vi "example_00_architecture.vi"() -> ()   [LabVIEW 2015, in "lv-recipe-machine.lvlib"]
uses:
  lv-recipe-machine.lvlib
  public/_controls/mode.ctl
  public/_controls/manual_state.ctl
  public/_controls/automatic_state.ctl
panel:
  out "step_elapsed_time":dbl
  out "recipe_elapsed_time":dbl
  out "automatic_state":T1
  out "manual_state":T2
  out "mode 2":T3
  out "step":string
  out "data":variant
  in  "mode":T3
  in  "update_mode":bool
  out "error out":errorcluster
  in  "stop":bool
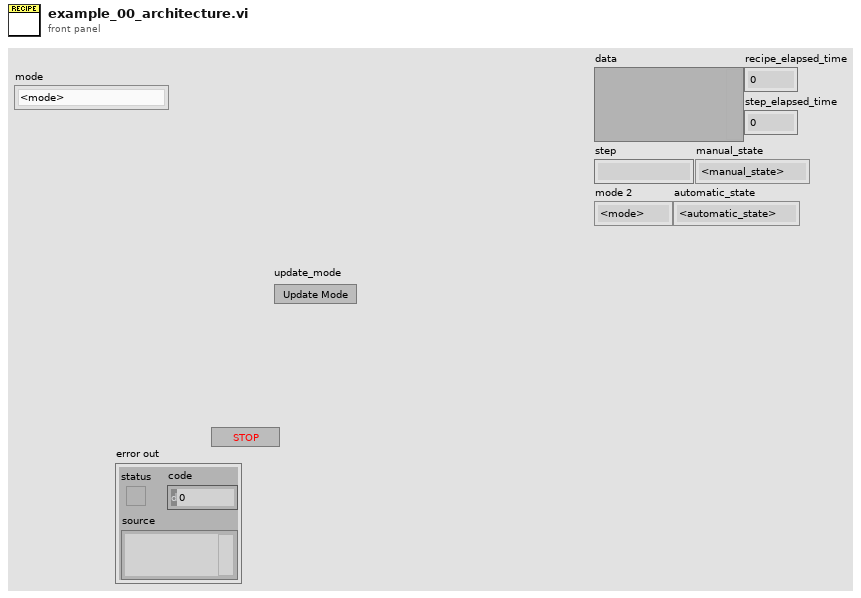
[diagram p1: front panel]
types:
  T1 = typedef "lv-recipe-machine.lvlib/automatic_state.ctl" = enum16{"<automatic_state>", "failed", "idle", "running", "paused", "stopped", "<null>"}
  T2 = typedef "lv-recipe-machine.lvlib/manual_state.ctl" = enum16{"<manual_state>", "failed", "action", "running", "idle", "<null>"}
  T3 = typedef "lv-recipe-machine.lvlib/mode.ctl" = enum16{"<mode>", "manual", "automatic", "<null>"}
  T4 = cluster{"change_out":refnum<event-registration>, "status_event_registration":refnum<event-registration>}
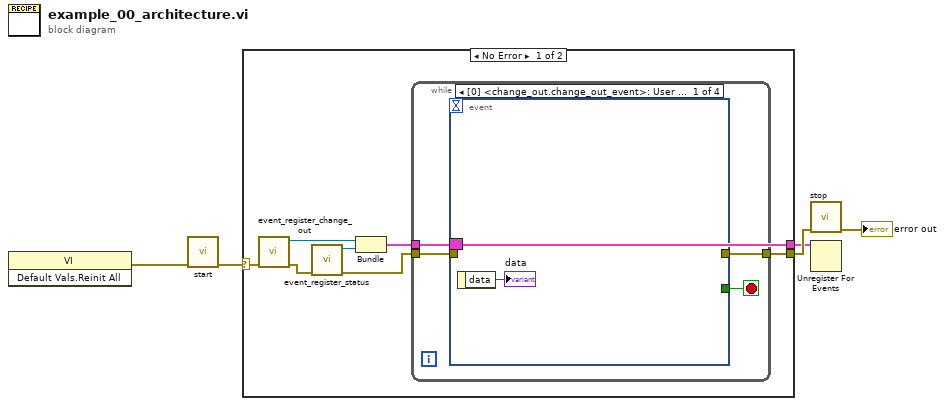
[diagram p0: block diagram]
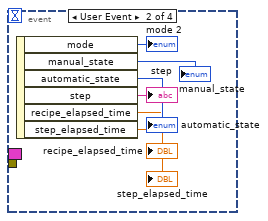
[diagram p2: hidden frame]
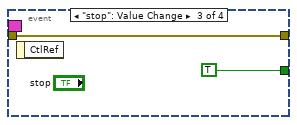
[diagram p3: hidden frame]
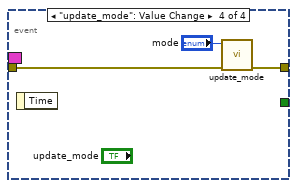
[diagram p4: hidden frame]
diagram:
  n1 = invoke class="VI" method="Default Vals.Reinit All"() -> (error out=w4:errorcluster)  [unwired: 3 in, 2 out]
  n2 = call "start.vi"("error in (no error)"=w4) -> ("error out"=w3:errorcluster)  [unwired: 10 in]
  n3 = case shown="No Error" w3 {
    selector: w3 -> [w8 w29]
    tunnel: [w12 w29] -> w5
    tunnel: [w9 _] -> w2
    frame No Error {
      n4 = call "event_register_change_out.vi"("error in (no error)"=w8) -> ("error out"=w7:errorcluster, "change_out"=w10:refnum<event-registration>)  [unwired: 9 in]
      n5 = call "event_register_status.vi"("error in (no error)"=w7) -> ("error out"=w6:errorcluster, "status_event_registration"=w11:refnum<event-registration>)  [unwired: 9 in]
      n6 = Bundle("change_out"=w10, "status_event_registration"=w11) -> (w9:T4)  [unwired: 1 in]
      n7 = while {
        tunnel: w6 -> [w16]
        tunnel: [w15] -> w12
        tunnel: w9 -> [w13]
        stop <- w14 stop-if-true
        n8 = event shown="[0] <change_out.change_out_event>: User Event" {
          selector: w13 -> [_ _ _ _]
          dyn-events: _ -> [_ _ _ _]
          timeout: _ -> [_ _ _ _]
          tunnel: w16 -> [_ _ w25 w27]
          tunnel: [_ _ w25 w28] -> w15
          tunnel: [_ _ TRUE _] -> w14
          event User Event {
            n9 = event-data() -> ("data"=→"data":variant)  [unwired: 1 in]
          }
          event User Event {
            n10 = event-data() -> ("mode"=→"mode 2":T3, "manual_state"=→"manual_state":T2, "automatic_state"=→"automatic_state":T1, "step"=→"step":string, "recipe_elapsed_time"=→"recipe_elapsed_time":dbl, "step_elapsed_time"=→"step_elapsed_time":dbl)  [unwired: 1 in]
          }
          event "stop": Value Change {
            n11 = event-data() -> ()  [unwired: 1 in, 1 out]
          }
          event "update_mode": Value Change {
            n12 = event-data() -> ()  [unwired: 1 in, 1 out]
            n13 = call "update_mode.vi"("error in (no error)"=w27, "mode"="mode") -> ("error out"=w28:errorcluster)  [unwired: 9 in]
          }
        }
      }
    }
    frame Error {
    }
  }
  n14 = call "stop.vi"("error in (no error)"=w5) -> ("error out"=→"error out":errorcluster)  [unwired: 10 in]
  n15 = Unregister For Events(event registration refnum=w2) -> ()  [unwired: 1 in, 1 out]
